vi "data queue.vi"(7 "Action":T1=enum."Enqueue", 8 "error in (no error)":errorcluster, 9 "timeout in ms (-1)":i32=10, 10 "data in":sgl[](array[numeric])) -> (0 "error out":errorcluster, 2 "data out":sgl[](array[numeric]), 3 "# elements in queue":i32, 11 "Empty?":bool)   [LabVIEW 2018]
uses:
  Queue Manager Actions.ctl
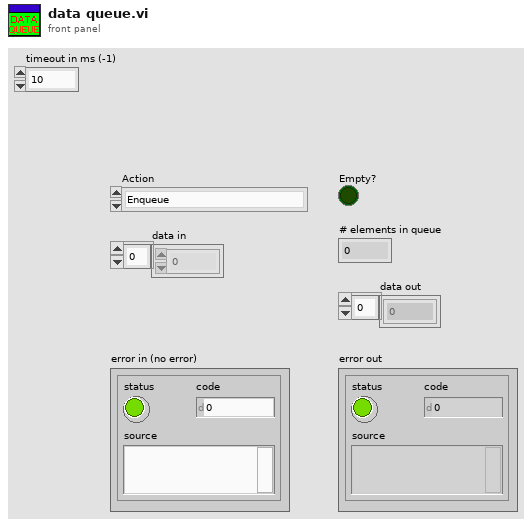
[diagram p1: front panel]
types:
  T1 = typedef "Queue Manager Actions.ctl" = enum16{"Init", "Enqueue", "Enqueue All", "Preview Queue", "Dequeue", "Get Status", "Flush Queue", "Flush All Queues", "Release All Queues", "Release Queue", "Enqueue at Opposite End"}
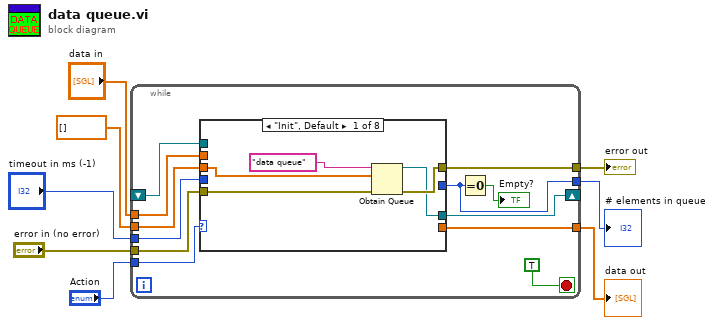
[diagram p0: block diagram]
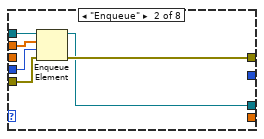
[diagram p2: hidden frame]
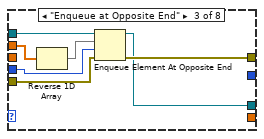
[diagram p3: hidden frame]
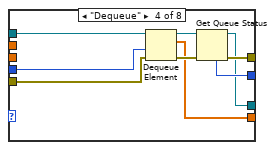
[diagram p4: hidden frame]
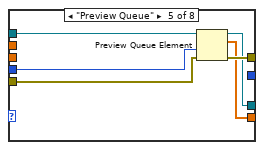
[diagram p5: hidden frame]
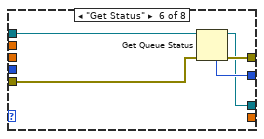
[diagram p6: hidden frame]
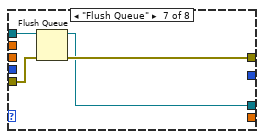
[diagram p7: hidden frame]
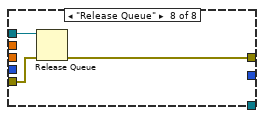
[diagram p8: hidden frame]
diagram:
  n1 = while {
    tunnel: "Action" -> [w16]
    tunnel: "error in (no error)" -> [w14]
    tunnel: [w20] -> w8
    shift-right: [w18] -> _
    shift-left: _ -> [w15]
    tunnel: "data in" -> [w13]
    tunnel: "timeout in ms (-1)" -> [w12]
    tunnel: [w11] -> w3
    tunnel: [w10] -> w2
    tunnel: sgl[] [] -> [w9]
    stop <- TRUE stop-if-true
    n2 = case shown="\"Init\", Default" w16 {
      tunnel: w15 -> [_ w27 w33 w42 w49 w55 w60 w63]
      tunnel: [w23 w30 w37 w45 w52 w57 w61 w64] -> w20
      tunnel: w14 -> [w24 w31 w38 w47 w53 w58 w62 w65]
      tunnel: [_ _ _ w41 w51 _ _ _] -> w11
      tunnel: [w21 w26 w32 w40 w48 w54 w59 _] -> w18
      tunnel: w12 -> [_ w29 w36 w39 w50 _ _ _]
      tunnel: [_ _ _ w43 _ w56 _ _] -> w10
      tunnel: w13 -> [_ w28 w35 _ _ _ _ _]
      tunnel: w9 -> [w22 _ _ _ _ _ _ _]
      frame "Init", Default {
        n3 = Obtain Queue(name (unnamed)="data queue", element data type=w22, error in (no error)=w24) -> (queue out=w21:refnum<queue>, error out=w23:errorcluster)  [unwired: 2 in, 1 out]
      }
      frame "Enqueue" {
        n4 = Enqueue Element(queue=w27, element=w28, timeout in ms (-1)=w29, error in (no error)=w31) -> (queue out=w26:refnum<queue>, error out=w30:errorcluster)  [unwired: 1 out]
      }
      frame "Enqueue at Opposite End" {
        n5 = Reverse 1D Array(array=w35) -> (reversed array=w34:sgl[])
        n6 = Enqueue Element At Opposite End(queue=w33, element=w34, timeout in ms (-1)=w36, error in (no error)=w38) -> (queue out=w32:refnum<queue>, error out=w37:errorcluster)  [unwired: 1 out]
      }
      frame "Dequeue" {
        n7 = Dequeue Element(queue=w42, timeout in ms (-1)=w39, error in (no error)=w47) -> (queue out=w44:refnum<queue>, element=w41:sgl[], error out=w46:errorcluster)  [unwired: 1 out]
        n8 = Get Queue Status(queue=w44, error in (no error)=w46) -> (queue out=w40:refnum<queue>, error out=w45:errorcluster, # elements in queue=w43:i32)  [unwired: 1 in, 5 out]
      }
      frame "Preview Queue" {
        n9 = Preview Queue Element(queue=w49, timeout in ms (-1)=w50, error in (no error)=w53) -> (queue out=w48:refnum<queue>, element=w51:sgl[], error out=w52:errorcluster)  [unwired: 1 out]
      }
      frame "Get Status" {
        n10 = Get Queue Status(queue=w55, error in (no error)=w58) -> (queue out=w54:refnum<queue>, error out=w57:errorcluster, # elements in queue=w56:i32)  [unwired: 1 in, 5 out]
      }
      frame "Flush Queue" {
        n11 = Flush Queue(queue=w60, error in (no error)=w62) -> (queue out=w59:refnum<queue>, error out=w61:errorcluster)  [unwired: 1 out]
      }
      frame "Release Queue" {
        n12 = Release Queue(queue=w63, error in (no error)=w65) -> (error out=w64:errorcluster)  [unwired: 1 in, 2 out]
      }
    }
    n13 = Equal To 0?(x=w10) -> (x = 0?=→"Empty?":bool)
  }
  "error out" <- w8
  "data out" <- w3
  "# elements in queue" <- w2
